vi "gyro -- async sweeper monitor V3.vi"(11 "sweeper monitor event pair":T4) -> ()   [LabVIEW 2021]
uses:
  filename-pattern.ctl
  show-win- control.ctl
  cursor winow.ctl
  server talk-to-back pair.ctl
  server talkback message type.ctl
  server talkto message type.ctl
  cursor window action.ctl
  launch items list.ctl
  que event bag action.ctl
  publisher action.ctl
  file -- read-write control.ctl
  array -- freq-voltage transformations action.ctl
  KM_file -- read-write control.ctl
  filename-action.ctl
  <vilib>/Analysis/baseanly.llb/A x B.vi
  <vilib>/Analysis/baseanly.llb/Complex A x B.vi
  Q -- check range -- i -- real.vi
  line -- complex.vi
  Q -- check range -- i -- integer.vi
  array -- freq-voltage transformations.vi/05c44075-957c-bc42-b6fa-2799d0bc0485.vi
  Q - not nan -- real.vi
  Q - not nan -- integer.vi
  <vilib>/Array/Sort 2D Array - Pop Stack.vi
  <vilib>/Array/Sort 2D Array - Push Stack.vi
  array -- freq-voltage transformations.vi/05c44075-957c-bc42-b6fa-2799d0bc0485.vi/269d4b3b-47f5-49e3-8884-44851e4dd9d5.vi
  array -- freq-voltage transformations.vi/05c44075-957c-bc42-b6fa-2799d0bc0485.vi/6d99389c-673d-4efb-bf33-19b32bcf4cf8.vi
  <vilib>/Analysis/Matrix/Numeric/Conversions/Array To Matrix.vi
  <vilib>/Analysis/Matrix/Numeric/Conversions/Array To Matrix - RA2.vi
  <vilib>/Analysis/baseanly.llb/Inverse Matrix.vi
  <vilib>/Analysis/baseanly.llb/Real Inverse Matrix.vi
panel:
  in  "sweeper panel":T1(tab)
  out "Plot: sweep window":cluster{"Freq out (Hz)":dbl[], dbl[]}[](graph)
  in  "!sweep :r":bool
  in  ":sweep is ON":bool
  in  "win":T2={"cen (Hz)"=41875.213593347406, "win (Hz)"=215.45804491715933, "left (Hz)"=41767.484570888824, "right (Hz)"=41982.94261580599}
  in  "subtract bgnd!":bool
  in  "fit!":bool=TRUE
  in  "cursor window":T3={"left"=41767.484570888824, "right "=41982.94261580599, "center"=41875.213593347406, "window"=215.45804491715933, "cursors"=[0, 1, 2], "relative"=0, "absolute"=0, "fixed vertical offset"=0.0, "vertical offset"=0.0, "skew"=0.0, "default window frac"=0.1, "kind"=enum."symmetric", "skew.left"=0.5, "skew.right"=0.5, "Plot ref"=refnum, "wing order"=enum."forw"}
  in  "async sweeper  engine event pair":T4
  in  "fitter event pair":T4
  in  "Read from file":path=path "/opt/new/Dropbox/In-nanocal-2021/Indium_June2021_035_0.8K_35T_sh_ark.dat"
  in  "Read from file :l":bool
  in  "tr":T5(ring)
  in  "save data":enum32{"save/read"}(tab)
  in  "Save to file :s":bool
  in  "Freq sweep name template":T6={"prefix"="RuCl3-rod", "group"="f"}
  in  "Save folder":path=path "/opt/data"
  in  "freq sweep file name":string="f004_RuCl3-rod_060221.dat"
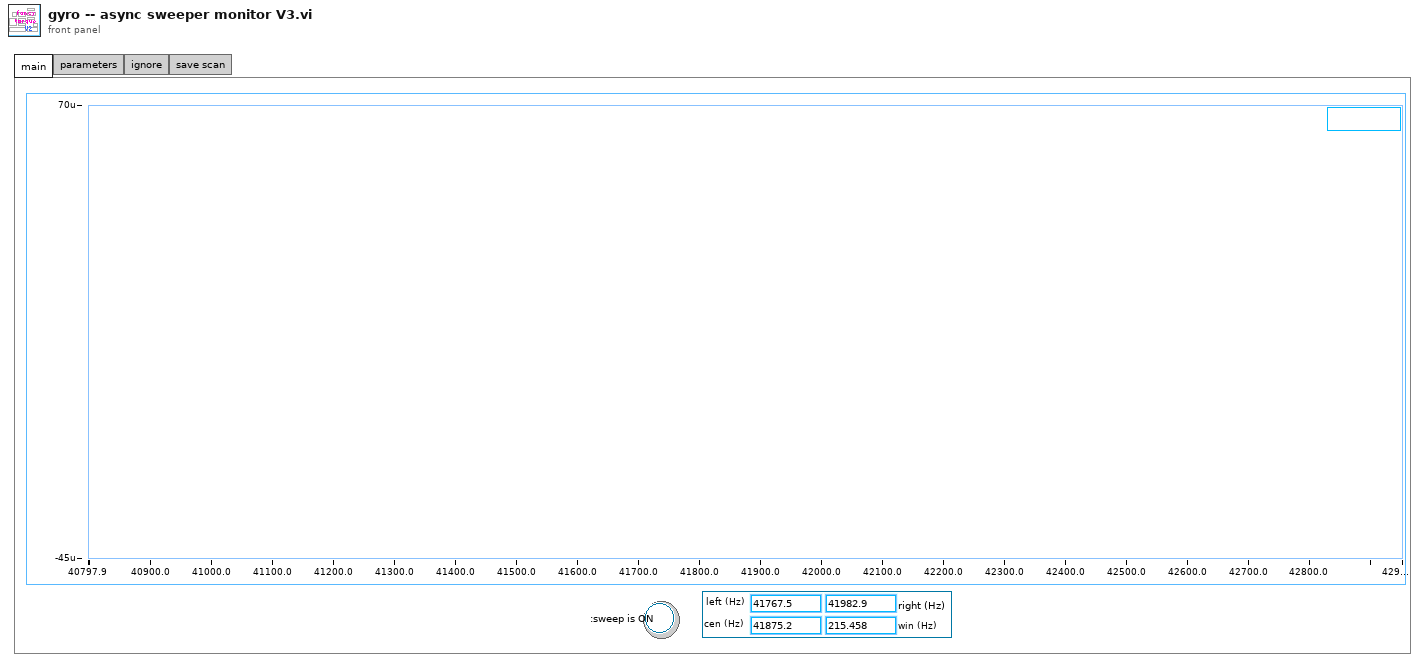
[diagram p1: front panel]
types:
  T1 = enum32{"main", "parameters", "ignore", "save scan"}
  T2 = typedef "show-win- control.ctl" = cluster{"cen (Hz)":dbl, "win (Hz)":dbl, "left (Hz)":dbl, "right (Hz)":dbl}
  T3 = typedef "cursor winow.ctl" = cluster{"left":dbl, "right ":dbl, "center":dbl, "window":dbl, "cursors":i32[], "relative":i32, "absolute":i32, "fixed vertical offset":dbl, "vertical offset":dbl, "skew":dbl, "default window frac":dbl, "kind":enum16{"symmetric", "skewed", "fancy"}, "skew.left":dbl, "skew.right":dbl, "Plot ref":refnum<vi>, "wing order":enum16{"forw", "back"}}
  T4 = typedef "server talk-to-back pair.ctl" = cluster{"talkback event":refnum<user-event>, "talkto event":refnum<user-event>}
  T5 = enum16{"as is", "add negative freq", "full rydh"}
  T6 = typedef "filename-pattern.ctl" = cluster{"prefix":string, "group":string}
  T7 = typedef "launch items list.ctl" = enum16{"source", "pll engine", "pll monitor", "sweeper engine", "sweeper monitor", "fitter"}
  T8 = typedef "que event bag action.ctl" = enum16{"check", "add", "init", "keys", "values"}
  T9 = typedef "cursor window action.ctl" = enum16{"balance", "h. offset change", "cursor moves", "change center", "change window", "init", "check", "reset", "set y to middle", "idle", "-write all Y", "-write left.X", "-write center.X", "-write right.X", "-write all X", "-change center", "-change window", "-change skew", "-read cursor 2", "-read cursor 1", "-read cursor 0", "-read all cursors", "-reset", "-read plot scale", "-set y to middle", "-Q: center.Y is visible", "-Q: window is visible", "-parse center.Y", "-right left from center", "-left move", "-right move", "-set center.Y", "-empty", "-set cursors to default", "-check", "-write center.Y", "-copy cursor 1", "-copy cursor 0", "-copy cursor 2", "move right", "move left", "shrink", "broaden", "skew up", "skew down", "-write plot scale", "zoom X", "change cen&win", "zoom to all data", "color--red", "color--green", "color--yellow", "read", "zoom out", "zoom in", "slide right", "slide left", "set range aspect ratio to 1", "move to window range", "--move to window range"}
  T10 = typedef "publisher action.ctl" = enum16{"set", "get", "init", "check"}
  T11 = typedef "file -- read-write control.ctl" = enum16{"read", "write all", "append one line"}
  T12 = typedef "array -- freq-voltage transformations action.ctl" = enum16{"as is", "add -ω", "sort ω", "2 x ω", "R-phase(deg) to Re-Im", "select ω>0", "labview file str", "select |ω|<max", "apply RC transform", "subtract background"}
  T13 = typedef "filename-action.ctl" = enum16{"rewrite", "parse", "force pattern", "uniquenum", "get T", "get B", "get ind", "get deg", "get name", "get folder", "get extension", "get basename", "get side", "get setof", "getID", "getIDStock", "remove prefix"}
  T14 = typedef "KM_file -- read-write control.ctl" = enum16{"read", "write all", "append one line"}
  T15 = typedef "server talkto message type.ctl" = cluster{"message":enum16{"stop", "start", "update pars", "update request", "new", "launch", "exit", "get", "reset", "pause", "unpause"}}
  T16 = typedef "eventvkey.ctl" = enum16{"ASCII", "Enter", "Return", "Shift", "Ctrl", "Alt", "Cmd", "Opt", "Caps", "NumLock", "Clear", "Break", "Up", "Down", "Left", "Right", "Insert", "Delete", "Home", "End", "PageUp", "PageDown", "Escape", "Help", "Pause", "ScrollLock", "F1", "F2", "F3", "F4", "F5", "F6", "F7", "F8", "F9", "F10", "F11", "F12", "F13", "F14", "F15", "F16", "F17", "F18", "F19", "F20", "F21", "F22", "F23", "F24", "Play", "VolumeUp", "VolumeDown", "Mute", "Two Byte Char"}
  T17 = enum16{"stop", "start", "update pars", "update request", "new", "launch", "exit", "get", "reset", "pause", "unpause"}
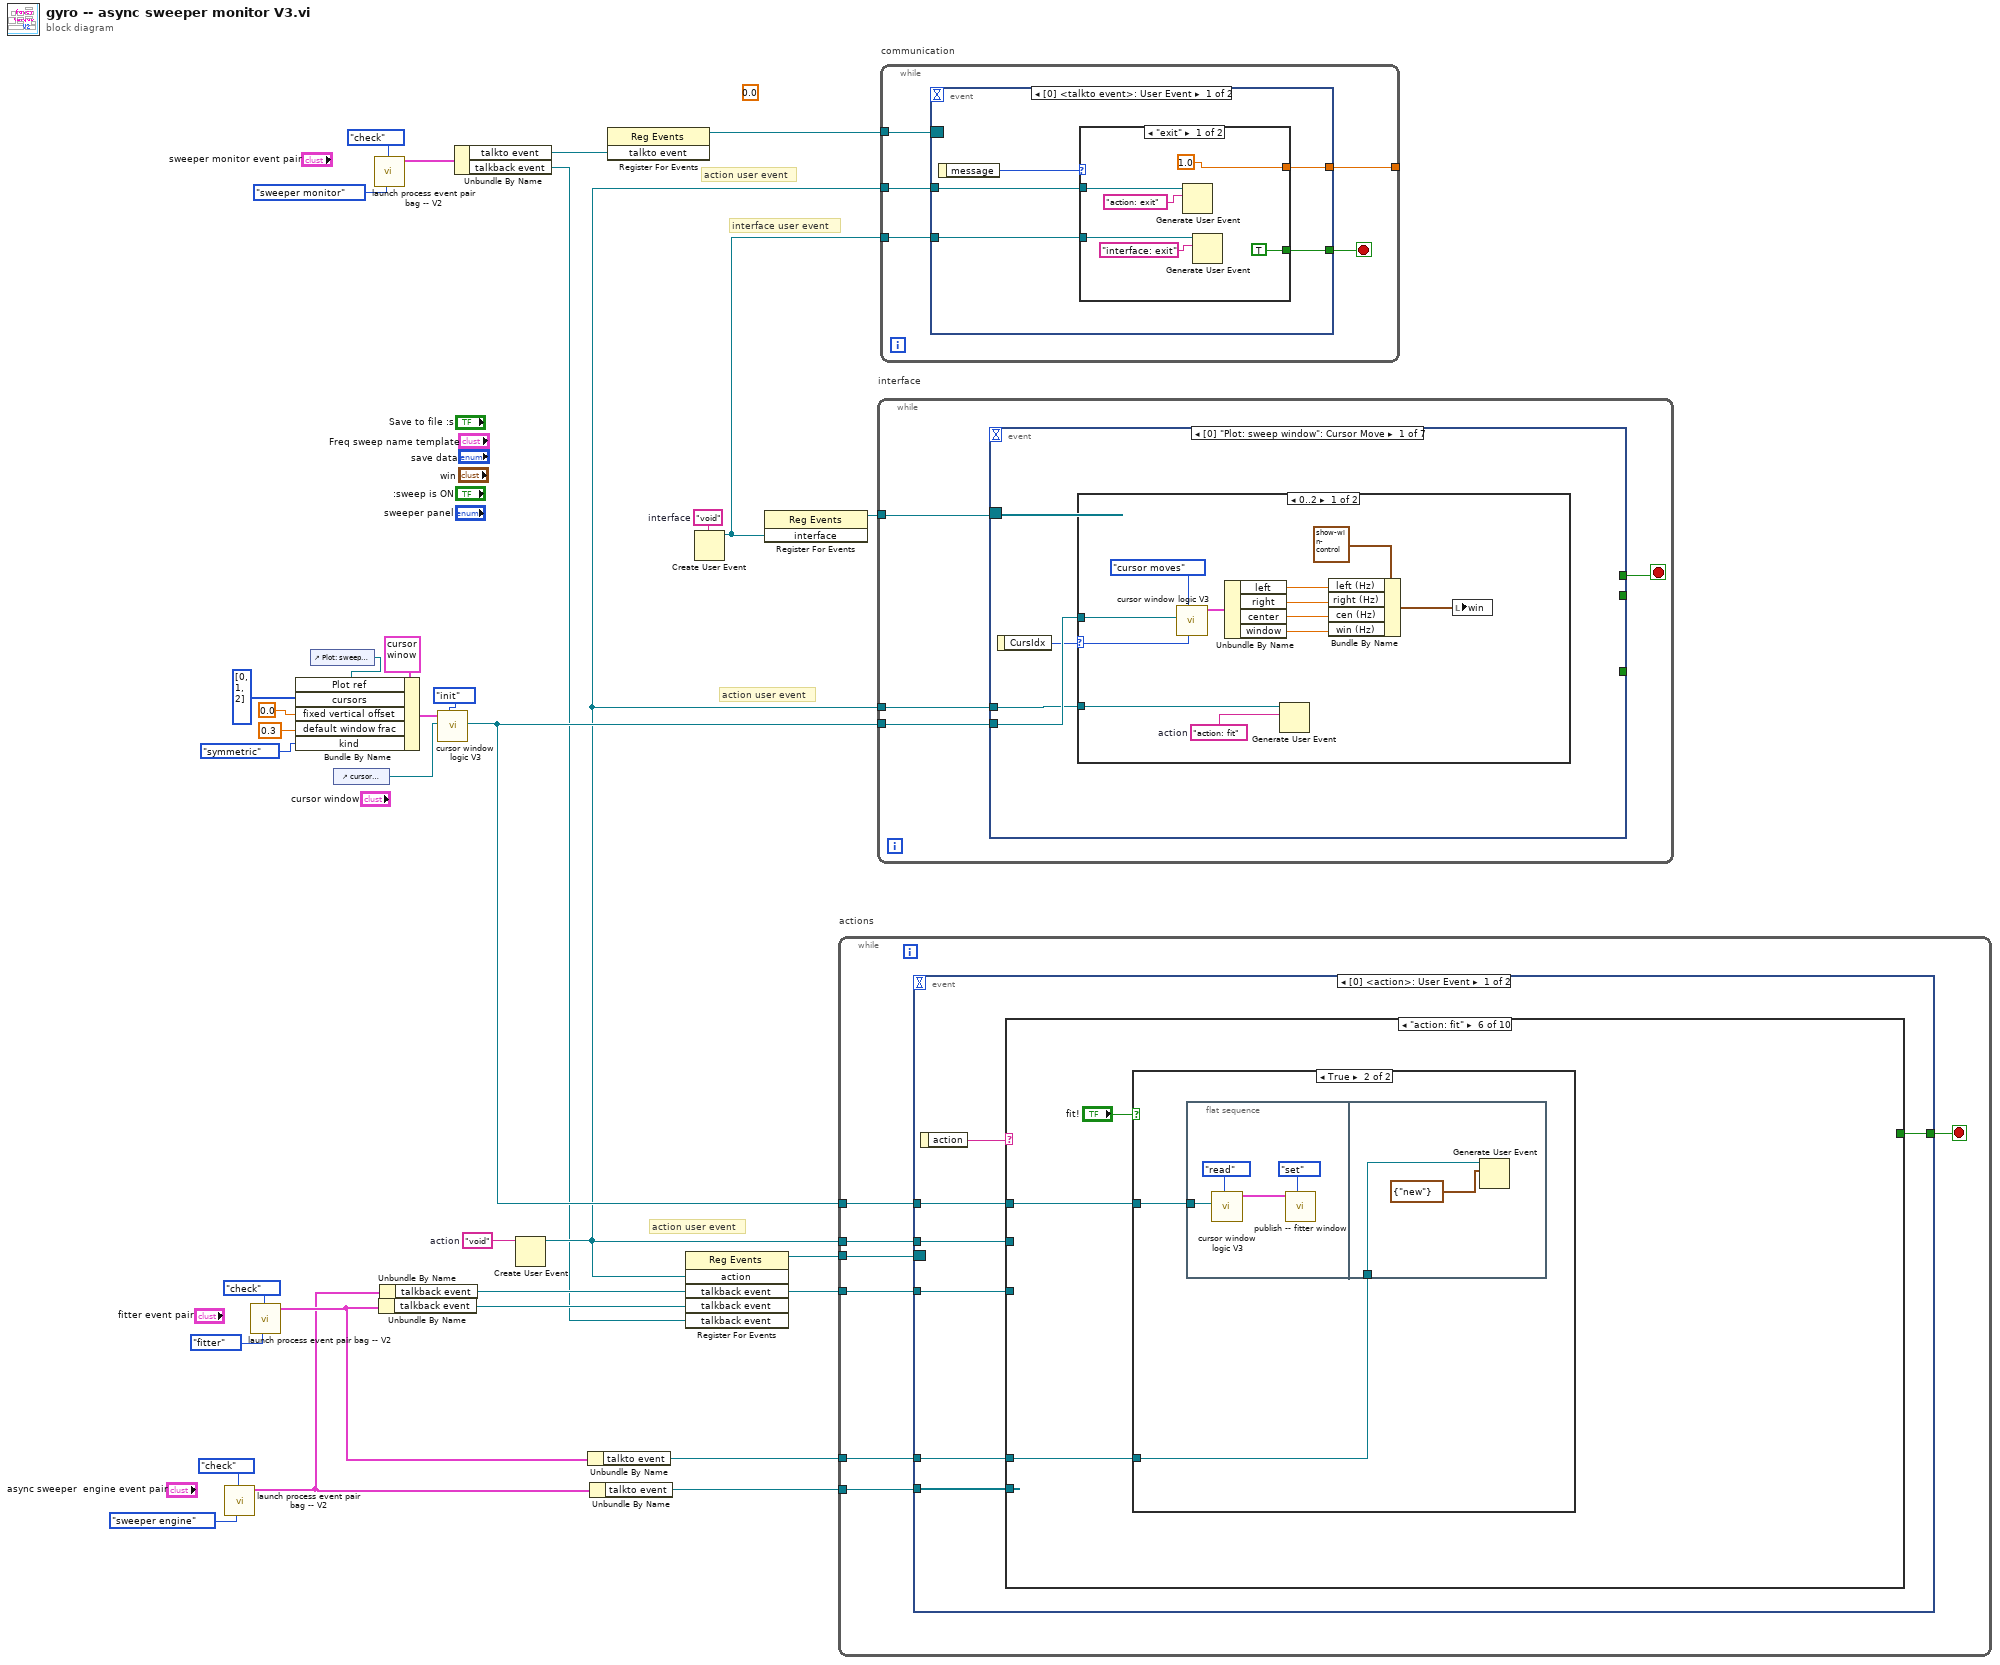
[diagram p0: block diagram]
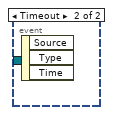
[diagram p3: hidden frame]
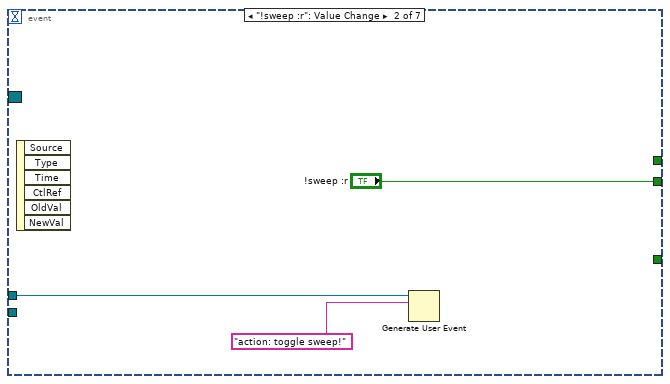
[diagram p5: hidden frame]
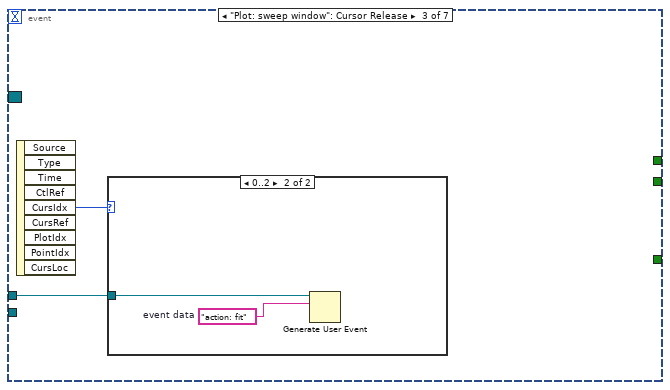
[diagram p6: hidden frame]
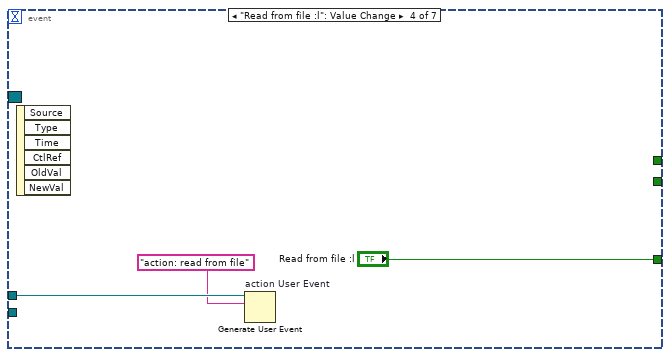
[diagram p8: hidden frame]
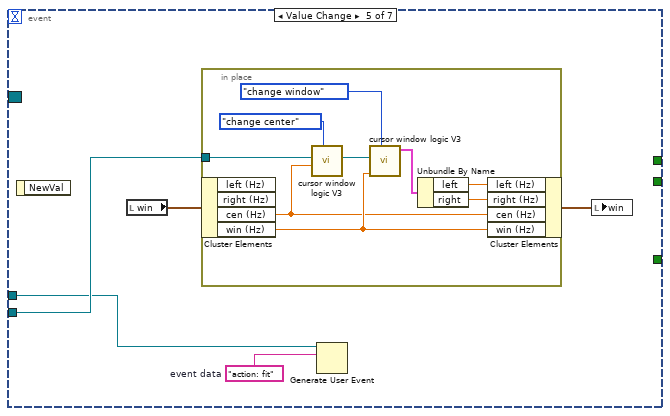
[diagram p9: hidden frame]
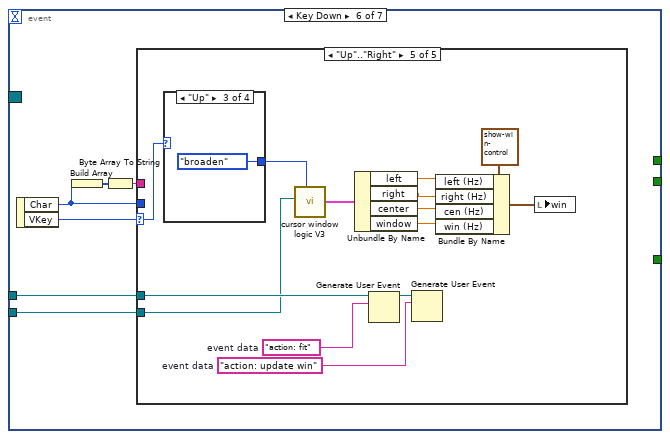
[diagram p10: hidden frame]
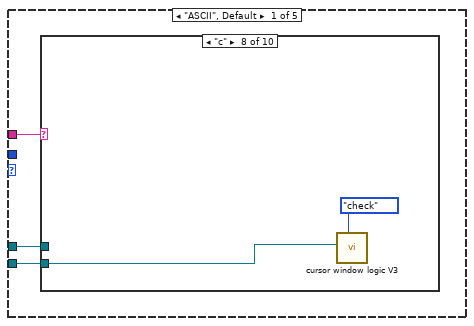
[diagram p11: hidden frame]
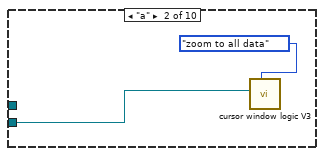
[diagram p13: hidden frame]
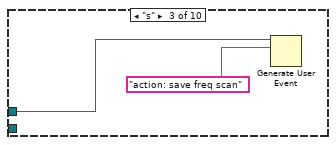
[diagram p14: hidden frame]
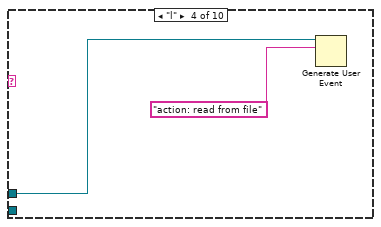
[diagram p15: hidden frame]
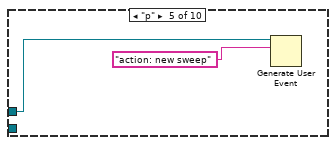
[diagram p16: hidden frame]
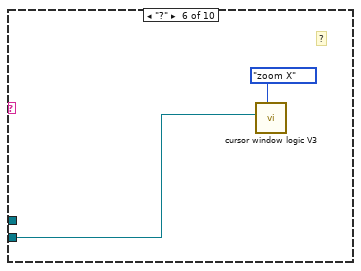
[diagram p17: hidden frame]
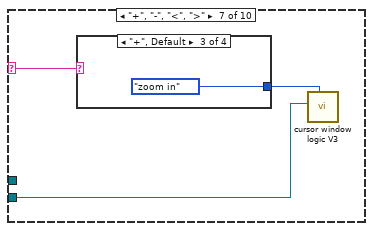
[diagram p18: hidden frame]
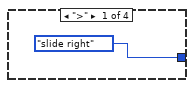
[diagram p19: hidden frame]
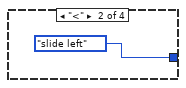
[diagram p20: hidden frame]
diagram:
  (unwired) 0.0 ("aaaaaa")
  w29 = "void"  # interface
  w31 = "void"  # action
  # "action user event"
  # "interface user event"
  # "action user event"
  # "action user event"
  n1 = call "launch process event pair bag -- V2.vi"("launch item"=launch_items_list."sweeper engine", "bag action"=que_event_bag_action."check") -> ("event pair OUT"=w4:T4)  [unwired: 7 in, 2 out]
  n2 = call "launch process event pair bag -- V2.vi"("launch item"=launch_items_list."fitter", "bag action"=que_event_bag_action."check") -> ("event pair OUT"=w7:T4)  [unwired: 7 in, 2 out]
  n3 = control-ref of="Plot: sweep window"() -> (w20:refnum<vi>)
  n4 = Bundle By Name(cluster=T3 {"left"=0.0, "right "=0.0, "center"=0.0, "window"=0.0, "cursors"=[], "relative"=0, "absolute"=0, "fixed vertical offset"=0.0, "vertical offset"=0.0, "skew"=0.0, "default window frac"=0.0, "kind"=enum."symmetric", "skew.left"=0.0, "skew.right"=0.0, "Plot ref"=refnum, "wing order"=enum."forw"} ("cursor bracket: All, data window"), "Plot ref"=w20, "cursors"=i32[] [0, 1, 2], "fixed vertical offset"=0.0, "default window frac"=0.3 ("fixed vertical offset"), "kind"=enum16{"symmetric", "skewed", "fancy"}."symmetric") -> (w24:T3)
  n5 = control-ref of="cursor window"() -> (w19:refnum<vi>)
  n6 = call "launch process event pair bag -- V2.vi"("launch item"=launch_items_list."sweeper monitor", "bag action"=que_event_bag_action."check") -> ("event pair OUT"=w1:T4)  [unwired: 7 in, 2 out]
  n7 = Unbundle By Name(w7) -> ("talkback event"=w16:refnum<user-event>)
  n8 = Unbundle By Name(w4) -> ("talkback event"=w15:refnum<user-event>)
  n9 = call "cursor window logic V3.vi"("cursor window action"=cursor_window_action."init", "cursor window in"=w19, "cursor window init"=w24) -> ("cursor window out"=w22:refnum<vi>)  [unwired: 7 in, 1 out]
  n10 = Unbundle By Name(w1) -> ("talkto event"=w13:refnum<user-event>, "talkback event"=w10:refnum<user-event>)
  n11 = Create User Event(user event datatype=w31) -> (user event=w11:refnum<user-event>)  [unwired: 1 in, 1 out]
  n12 = Unbundle By Name(w7) -> ("talkto event"=w17:refnum<user-event>)
  n13 = Unbundle By Name(w4) -> ("talkto event"=w18:refnum<user-event>)
  n14 = register-events(w13) -> (reference out=w14:refnum<event-registration>)  [unwired: 2 in, 1 out]
  n15 = register-events(w11, w15, w16, w10) -> (reference out=w32:refnum<event-registration>)  [unwired: 2 in, 1 out]
  n16 = Create User Event(user event datatype=w29) -> (user event=w12:refnum<user-event>)  [unwired: 1 in, 1 out]
  n17 = register-events(w12) -> (reference out=w30:refnum<event-registration>)  [unwired: 2 in, 1 out]
  n18 = while "actions" {
    tunnel: w32 -> [w39]
    tunnel: w11 -> [w38]
    tunnel: w22 -> [w37]
    tunnel: w18 -> [w36]
    tunnel: w15 -> [w35]
    tunnel: w17 -> [w34]
    stop <- w33 stop-if-true
    n19 = event shown="[0] <action>: User Event" {
      selector: w39 -> [_ _]
      dyn-events: _ -> [_ _]
      timeout: _ -> [_ _]
      tunnel: w38 -> [w45 w169]
      tunnel: w37 -> [w44 _]
      tunnel: w36 -> [w43 _]
      tunnel: w35 -> [w42 _]
      tunnel: w34 -> [w41 _]
      tunnel: [w40 _] -> w33
      event User Event {
        n20 = event-data() -> ("action"=w46:string)  [unwired: 1 in]
        n21 = case shown="\"action: fit\"" w46 {
          tunnel: w45 -> [w55 w80 _ w88 _ _ _ _ _ _]
          tunnel: w44 -> [_ _ _ _ _ w146 _ _ _ _]
          tunnel: w43 -> [_ _ _ _ _ _ w159 w164 w168 _]
          tunnel: w42 -> [_ _ _ _ _ _ _ _ _ _]
          tunnel: w41 -> [_ _ _ _ _ w144 _ _ _ _]
          tunnel: [_ _ TRUE _ _ _ _ _ _ _] -> w40
          frame "action: new sweep" {
            n22 = call "MFLI -- publish -- freq scan.vi"("publisher action"=publisher_action."get") -> ("Voltage out (V)"=w52:cdb[], "Freq out (Hz)"=w54:dbl[])  [unwired: 9 in]
            n23 = case shown="True" "subtract bgnd!" {
              tunnel: w54 -> [w67 w75]
              tunnel: [w61 w75] -> w53
              tunnel: w52 -> [w63 w74]
              tunnel: [w68 w74] -> w51
              frame True {
                w60 = 10 ("length")
                n24 = Delete From Array(array=w67, length=w60, index=0) -> (array with subset deleted=w66:dbl[])  [unwired: 1 out]
                n25 = Delete From Array(array=w63, length=w60, index=0) -> (array with subset deleted=w62:cdb[])  [unwired: 1 out]
                n26 = call "linear interp iiii- complex - z-omega.vi"("z"=w62, "omega"=w66) -> ("z out"=w69:cdb[], "omega out"=w61:dbl[], "intercept"=w71:cdb, "slope"=w72:cdb)  [unwired: 5 in, 5 out]
                n27 = Multiply(x=w61, y=w72) -> (x*y=w73:cdb[])
                n28 = Add(x=w73, y=w71) -> (x+y=w70:cdb[])
                n29 = Subtract(x=w69, y=w70) -> (x-y=w68:cdb[])
              }
              frame False {
              }
            }
            n30 = Generate User Event(user event=w55, event data cluster="action: fit" ("event data")) -> ()  [unwired: 2 in, 2 out]
            n31 = Complex To Re/Im(x + iy=w51) -> (x=w58:dbl[], y=w57:dbl[])
            n32 = Bundle("Freq out (Hz)"=w53, w58) -> (w59:cluster{"Freq out (Hz)":dbl[], dbl[]})  [unwired: 1 in]
            n33 = Bundle("Freq out (Hz)"=w53, w57) -> (w56:cluster{"Freq out (Hz)":dbl[], dbl[]})  [unwired: 1 in]
            n34 = Build Array(w59, w56) -> (→"Plot: sweep window":cluster{"Freq out (Hz)":dbl[], dbl[]}[])
          }
          frame "action: toggle sweep!" {
            n35 = local read ":sweep is ON"() -> (w79:bool)
            n36 = Select(t="action: stop sweep!" ("event data"), s=w79, f="action: start sweep!" ("event data")) -> (s? t:f=w76:string)
            n37 = Generate User Event(user event=w80, event data cluster=w76) -> ()  [unwired: 2 in, 2 out]
          }
          frame "action: exit" {
            n38 = local write ":sweep is ON"(FALSE ("sweep ON")) -> ()
          }
          frame "action: read from file" {
            n39 = disable-structure shown="Disabled" {
              frame Disabled {
                n40 = Fract/Exp String To Number(offset=u32 0 ("offset past scan")) -> ()  [unwired: 3 in, 2 out]
                n41 = Fract/Exp String To Number() -> ()  [unwired: 4 in, 2 out]
                n42 = Fract/Exp String To Number() -> ()  [unwired: 4 in, 2 out]
              }
              frame Enabled {
              }
            }
            n43 = call "file - read-write - list of lines.vi"("read/write control"=file_--_read-write_control."read", "file path"="Read from file") -> ("list of lines OUT"=w92:string[])  [unwired: 7 in, 2 out]
            n44 = for {
              tunnel: w92 -> [w128] mode=indexing
              tunnel: [w123] -> w87 mode=indexing if=w119
              tunnel: [w122] -> w86 mode=indexing if=w119
              w124 = 0.0
              n45 = Scan From String(format string="%f%f%f", input string=w128, initial scan location=u32 0, default 1=w124, default 2=w124, default 3=w124) -> (offset past scan=w120:u32, output 1=w122:dbl, output 2=w126:dbl, output 3=w125:dbl)  [unwired: 1 in, 2 out]
              n46 = Greater Than 0?(x=w120) -> (x > 0?=w119:bool)
              n47 = Re/Im To Complex(1:w125, 2:w126) -> (0:w123:cdb)
            }
            n48 = case shown="\"add negative freq\"" "tr" {
              tunnel: w87 -> [w95 w97 w109]
              tunnel: w86 -> [w96 w104 w118]
              tunnel: [w96 w101 w115] -> w84
              tunnel: [w95 w100 w114] -> w83
              frame "as is", Default {
              }
              frame "add negative freq" {
                n49 = call "array -- freq-voltage transformations.vi"("freq voltage action"=array_--_freq-voltage_transformations_action."add -ω", "z In"=w97, "ω IN"=w104) -> ("z out"=w102:cdb[], "ω out"=w103:dbl[])  [unwired: 5 in, 2 out]
                n50 = call "array -- freq-voltage transformations.vi"("freq voltage action"=array_--_freq-voltage_transformations_action."sort ω", "z In"=w102, "ω IN"=w103) -> ("z out"=w100:cdb[], "ω out"=w101:dbl[])  [unwired: 5 in, 2 out]
              }
              frame "full rydh" {
                n51 = call "array -- freq-voltage transformations.vi"("freq voltage action"=array_--_freq-voltage_transformations_action."2 x ω", "z In"=w109, "ω IN"=w118) -> ("z out"=w108:cdb[], "ω out"=w111:dbl[])  [unwired: 5 in, 2 out]
                n52 = call "array -- freq-voltage transformations.vi"("freq voltage action"=array_--_freq-voltage_transformations_action."R-phase(deg) to Re-Im", "z In"=w108, "ω IN"=w111) -> ("z out"=w107:cdb[], "ω out"=w110:dbl[])  [unwired: 5 in, 2 out]
                n53 = call "array -- freq-voltage transformations.vi"("freq voltage action"=array_--_freq-voltage_transformations_action."add -ω", "z In"=w107, "ω IN"=w110) -> ("z out"=w116:cdb[], "ω out"=w117:dbl[])  [unwired: 5 in, 2 out]
                n54 = call "array -- freq-voltage transformations.vi"("freq voltage action"=array_--_freq-voltage_transformations_action."sort ω", "z In"=w116, "ω IN"=w117) -> ("z out"=w114:cdb[], "ω out"=w115:dbl[])  [unwired: 5 in, 2 out]
              }
            }
            n55 = flat-sequence {
              tunnel: w88 -> [w132]
              tunnel: [w132] -> w93
              tunnel: w83 -> [w130]
              tunnel: w84 -> [w129]
              tunnel: w93 -> [w134]
              tunnel: "action: new sweep" ("event data") -> [w133]
              frame #0 {
                n56 = call "MFLI -- publish -- freq scan.vi"("publisher action"=publisher_action."set", "Voltage IN (V)"=w130, "Freq IN (Hz)"=w129) -> ()  [unwired: 7 in, 2 out]
              }
              frame #1 {
                n57 = Generate User Event(user event=w134, event data cluster=w133) -> ()  [unwired: 2 in, 2 out]
              }
            }
          }
          frame "action: save freq scan" {
            n58 = local read "Freq sweep name template"() -> (w140:T6)
            n59 = call "MFLI -- publish -- freq scan.vi"("publisher action"=publisher_action."get") -> ("Voltage out (V)"=w136:cdb[], "Freq out (Hz)"=w137:dbl[])  [unwired: 9 in]
            n60 = call "filename-manage.vi"("filename pattern"=w140, "filename-action"=filename-action."uniquenum", "folder IN"="Save folder", "file name IN"="freq sweep file name") -> ("filename OUT"=w139:string)  [unwired: 5 in, 2 out]
            n61 = call "KM_appendline -- freq sweep.vi"("freq"=w137, "Vout(V)"=w136, "Save frequency scan"="Save folder", "read/write control"=KM_file_--_read-write_control."append one line", "name or relative path"=w139) -> ()  [unwired: 15 in]
            n62 = local write "freq sweep file name"(w139) -> ()
          }
          frame "action: fit" {
            n63 = case shown="True" "fit!" {
              tunnel: w146 -> [_ w148]
              tunnel: w144 -> [_ w147]
              frame False {
              }
              frame True {
                n64 = flat-sequence {
                  tunnel: w148 -> [w151]
                  tunnel: w147 -> [w153]
                  frame #0 {
                    n65 = call "cursor window logic V3.vi"("cursor window action"=cursor_window_action."read", "cursor window in"=w151) -> ("cursor window out"=w150:T3)  [unwired: 8 in, 1 out]
                    n66 = call "publish -- fitter window.vi"("publisher action"=publisher_action."set", "win IN"=w150) -> ()  [unwired: 9 in, 1 out]
                  }
                  frame #1 {
                    n67 = Generate User Event(user event=w153, event data cluster=T15 {"message"=enum."new"} ("event data")) -> ()  [unwired: 2 in, 2 out]
                  }
                }
              }
            }
          }
          frame "action: start sweep!" {
            n68 = local read "win"() -> (w156:T2)
            n69 = call "publish -- sweeper window.vi"("publisher action"=publisher_action."set", "win IN"=w156) -> ()  [unwired: 9 in, 1 out]
            n70 = local write ":sweep is ON"(TRUE ("sweep ON")) -> ()
            n71 = Generate User Event(user event=w159, event data cluster=T15 {"message"=enum."update request"} ("event data")) -> (user event out=w158:refnum<user-event>)  [unwired: 2 in, 1 out]
            n72 = Generate User Event(user event=w158, event data cluster=T15 {"message"=enum."start"} ("event data")) -> ()  [unwired: 2 in, 2 out]
          }
          frame "action: stop sweep!" {
            n73 = Generate User Event(user event=w164, event data cluster=T15 {"message"=enum."stop"} ("event data")) -> ()  [unwired: 2 in, 2 out]
            n74 = local write ":sweep is ON"(FALSE ("sweep ON")) -> ()
          }
          frame "action: update win" {
            n75 = local read "win"() -> (w165:T2)
            n76 = call "publish -- sweeper window.vi"("publisher action"=publisher_action."set", "win IN"=w165) -> ()  [unwired: 9 in, 1 out]
            n77 = Generate User Event(user event=w168, event data cluster=T15 {"message"=enum."update request"} ("event data")) -> ()  [unwired: 2 in, 2 out]
          }
          frame "void", Default {
          }
        }
      }
      event User Event {
        n78 = event-data() -> ("message"=w170:enum16{"new", "void"})  [unwired: 1 in, 4 out]
        n79 = case shown="\"new\"" w170 {
          tunnel: w169 -> [w171 _]
          frame "new" {
            n80 = Generate User Event(user event=w171, event data cluster="action: new sweep" ("event data")) -> ()  [unwired: 2 in, 2 out]
          }
          frame "void", Default {
          }
        }
      }
    }
  }
  n81 = while "interface" {
    tunnel: w30 -> [w176]
    tunnel: w11 -> [w175]
    tunnel: w22 -> [w174]
    stop <- w173 stop-if-true
    n82 = event shown="[0] \"Plot: sweep window\": Cursor Move" {
      selector: w176 -> [_ _ _ _ _ _ _]
      dyn-events: _ -> [_ _ _ _ _ _ _]
      timeout: _ -> [_ _ _ _ _ _ _]
      tunnel: w175 -> [w177 w194 w196 w201 w202 w220 _]
      tunnel: w174 -> [w179 _ _ _ w206 w216 _]
      tunnel: [_ "!sweep :r" _ _ _ _ _] -> _
      tunnel: [_ _ _ "Read from file :l" _ _ _] -> _
      tunnel: [_ _ _ _ _ _ w264] -> w173
      event "Plot: sweep window": Cursor Move {
        n83 = event-data() -> ("CursIdx"=w178:i32)  [unwired: 1 in]
        n84 = case shown="0..2" w178 {
          selector: w178 -> [w189 _]
          tunnel: w179 -> [w191 _]
          tunnel: w177 -> [w187 _]
          frame 0..2 {
            w186 = "action: fit"  # action
            n85 = call "cursor window logic V3.vi"("CursIdx"=w189, "cursor window action"=cursor_window_action."cursor moves", "cursor window in"=w191) -> ("cursor window out"=w188:T3)  [unwired: 7 in, 1 out]
            n86 = Unbundle By Name(w188) -> ("left"=w183:dbl, "right"=w182:dbl, "center"=w181:dbl, "window"=w180:dbl)
            n87 = Generate User Event(user event=w187, event data cluster=w186) -> ()  [unwired: 2 in, 2 out]
            n88 = Bundle By Name(cluster=T2 {"cen (Hz)"=-0.35260838541595674, "win (Hz)"=17.234446484426172, "left (Hz)"=-8.969831627629043, "right (Hz)"=8.26461485679713} ("win"), "left (Hz)"=w183, "right (Hz)"=w182, "cen (Hz)"=w181, "win (Hz)"=w180) -> (w184:T2)
            n89 = local write "win"(w184) -> ()
          }
          frame 3..5, Default {
          }
        }
      }
      event "!sweep :r": Value Change {
        n90 = event-data() -> ()  [unwired: 1 in, 6 out]
        n91 = Generate User Event(user event=w194, event data cluster="action: toggle sweep!" ("event data")) -> ()  [unwired: 2 in, 2 out]
      }
      event "Plot: sweep window": Cursor Release {
        n92 = event-data() -> ("CursIdx"=w195:i32)  [unwired: 1 in, 8 out]
        n93 = case shown="0..2" w195 {
          tunnel: w196 -> [_ w197]
          frame 3, Default {
          }
          frame 0..2 {
            w198 = "action: fit"  # event data
            n94 = Generate User Event(user event=w197, event data cluster=w198) -> ()  [unwired: 2 in, 2 out]
          }
        }
      }
      event "Read from file :l": Value Change {
        n95 = event-data() -> ()  [unwired: 1 in, 6 out]
        n96 = Generate User Event "action User Event"(user event=w201, event data cluster="action: read from file" ("event data")) -> ()  [unwired: 2 in, 2 out]
      }
      event Value Change {
        w203 = "action: fit"  # event data
        n97 = event-data() -> ()  [unwired: 1 in, 1 out]
        n98 = local read "win"() -> (w205:T2)
        n99 = in-place {
          in-place-border: w206 -> [w212]
          n100 = in-place-cluster #1(w205) -> ("cen (Hz)"=w207:dbl, "win (Hz)"=w208:dbl)  [unwired: 2 out]
          n101 = call "cursor window logic V3.vi"("cursor window action"=cursor_window_action."change center", "center"=w207, "cursor window in"=w212) -> ("cursor window out"=w213:refnum<vi>)  [unwired: 7 in, 1 out]
          n102 = call "cursor window logic V3.vi"("cursor window action"=cursor_window_action."change window", "window"=w208, "cursor window in"=w213) -> ("cursor window out"=w211:T3)  [unwired: 7 in, 1 out]
          n103 = Unbundle By Name(w211) -> ("left"=w210:dbl, "right"=w209:dbl)
          n104 = in-place-cluster #1("left (Hz)"=w210, "right (Hz)"=w209, "cen (Hz)"=w207, "win (Hz)"=w208) -> (w204:T2)
        }
        n105 = Generate User Event(user event=w202, event data cluster=w203) -> ()  [unwired: 2 in, 2 out]
        n106 = local write "win"(w204) -> ()
      }
      event Key Down {
        n107 = event-data() -> ("Char"=w218:i16, "VKey"=w221:T16)  [unwired: 1 in]
        n108 = Build Array(w218) -> (w219:i16[])
        n109 = Byte Array To String(unsigned byte array=w219) -> (string=w217:string)
        n110 = case shown="\"Up\"..\"Right\"" w221 {
          selector: w221 -> [_ _ _ _ w259]
          tunnel: w218 -> [_ _ _ _ _]
          tunnel: w220 -> [w224 _ _ _ w258]
          tunnel: w217 -> [w223 _ _ _ _]
          tunnel: w216 -> [w222 _ _ _ w255]
          frame "ASCII", Default {
            n111 = case shown="\"c\"" w223 {
              selector: w223 -> [_ _ _ _ _ _ w236 _ _ _]
              tunnel: w224 -> [_ _ w227 w229 w231 _ _ _ _ w245]
              tunnel: w222 -> [_ w225 _ _ _ w233 w237 w242 _ _]
              frame "0", Default {
              }
              frame "a" {
                n112 = call "cursor window logic V3.vi"("cursor window action"=cursor_window_action."zoom to all data", "cursor window in"=w225) -> ()  [unwired: 8 in, 2 out]
              }
              frame "s" {
                n113 = Generate User Event(user event=w227, event data cluster="action: save freq scan" ("event data")) -> ()  [unwired: 2 in, 2 out]
              }
              frame "l" {
                n114 = Generate User Event(user event=w229, event data cluster="action: read from file" ("event data")) -> ()  [unwired: 2 in, 2 out]
              }
              frame "p" {
                n115 = Generate User Event(user event=w231, event data cluster="action: new sweep" ("event data")) -> ()  [unwired: 2 in, 2 out]
              }
              frame "?" {
                # "?"
                n116 = call "cursor window logic V3.vi"("cursor window action"=cursor_window_action."zoom X", "cursor window in"=w233) -> ()  [unwired: 8 in, 2 out]
              }
              frame "+", "-", "<", ">" {
                n117 = case shown="\"+\", Default" w236 {
                  tunnel: [cursor_window_action."slide right" ("cursor window action") cursor_window_action."slide left" ("cursor window action") cursor_window_action."zoom in" ("cursor window action") cursor_window_action."zoom out" ("cursor window action")] -> w235
                  frame ">" {
                  }
                  frame "<" {
                  }
                  frame "+", Default {
                  }
                  frame "-" {
                  }
                }
                n118 = call "cursor window logic V3.vi"("cursor window action"=w235, "cursor window in"=w237) -> ()  [unwired: 8 in, 2 out]
              }
              frame "c" {
                n119 = call "cursor window logic V3.vi"("cursor window action"=cursor_window_action."check", "cursor window in"=w242) -> ()  [unwired: 8 in, 2 out]
              }
              frame "t" {
              }
              frame "r" {
                n120 = Generate User Event(user event=w245, event data cluster="action: toggle sweep!" ("event data")) -> ()  [unwired: 2 in, 2 out]
              }
            }
          }
          frame "Escape" {
          }
          frame "PageUp" {
          }
          frame "PageDown" {
          }
          frame "Up".."Right" {
            w246 = "action: update win"  # event data
            w248 = "action: fit"  # event data
            n121 = case shown="\"Up\"" w259 {
              tunnel: [cursor_window_action."move right" ("cursor window action") cursor_window_action."move left" ("cursor window action") cursor_window_action."broaden" ("cursor window action") cursor_window_action."shrink" ("cursor window action")] -> w257
              frame "Right", Default {
              }
              frame "Left" {
              }
              frame "Up" {
              }
              frame "Down" {
              }
            }
            n122 = call "cursor window logic V3.vi"("cursor window action"=w257, "cursor window in"=w255) -> ("cursor window out"=w256:T3)  [unwired: 8 in, 1 out]
            n123 = Unbundle By Name(w256) -> ("left"=w252:dbl, "right"=w251:dbl, "center"=w250:dbl, "window"=w249:dbl)
            n124 = Generate User Event(user event=w258, event data cluster=w248) -> (user event out=w247:refnum<user-event>)  [unwired: 2 in, 1 out]
            n125 = Generate User Event(user event=w247, event data cluster=w246) -> ()  [unwired: 2 in, 2 out]
            n126 = Bundle By Name(cluster=T2 {"cen (Hz)"=-0.35260838541595674, "win (Hz)"=17.234446484426172, "left (Hz)"=-8.969831627629043, "right (Hz)"=8.26461485679713} ("win"), "left (Hz)"=w252, "right (Hz)"=w251, "cen (Hz)"=w250, "win (Hz)"=w249) -> (w254:T2)
            n127 = local write "win"(w254) -> ()
          }
        }
      }
      event User Event {
        n128 = event-data() -> ("interface"=w265:string)  [unwired: 1 in, 4 out]
        n129 = case shown="\"False\", Default" w265 {
          tunnel: [_ TRUE] -> w264
          frame "False", Default {
          }
          frame "interface: exit" {
          }
        }
      }
    }
  }
  n130 = while "communication" {
    tunnel: w14 -> [w271]
    tunnel: w11 -> [w269]
    tunnel: w12 -> [w268]
    tunnel: [w267] -> _
    stop <- w270 stop-if-true
    n131 = event shown="[0] <talkto event>: User Event" {
      selector: w271 -> [_ _]
      dyn-events: _ -> [_ _]
      timeout: _ -> [_ _]
      tunnel: [w275 _] -> w270
      tunnel: w269 -> [w274 _]
      tunnel: w268 -> [w273 _]
      tunnel: [w272 _] -> w267
      event User Event {
        n132 = event-data() -> ("message"=w276:T17)  [unwired: 1 in]
        n133 = case shown="\"exit\"" w276 {
          tunnel: [TRUE _] -> w275
          tunnel: w274 -> [w281 _]
          tunnel: w273 -> [w278 _]
          tunnel: [1.0 ("aaaaaa") _] -> w272
          frame "exit" {
            n134 = Generate User Event(user event=w281, event data cluster="action: exit" ("event data")) -> ()  [unwired: 2 in, 2 out]
            n135 = Generate User Event(user event=w278, event data cluster="interface: exit" ("event data")) -> ()  [unwired: 2 in, 2 out]
          }
          frame "start", Default {
          }
        }
      }
      event Timeout {
        n136 = event-data() -> ()  [unwired: 1 in, 3 out]
      }
    }
  }
